vi "Init.vi"() -> (3 "Template Msg Strategy out":refnum<class "Template Msg Strategy.lvclass">)   [LabVIEW 2021, in "jettl Msg Template.lvlib" / "Template Msg Strategy.lvclass"]
uses:
  Template Msg Strategy.lvclass
  Template Msg Strategy.lvclass/Template Msg Strategy.ctl
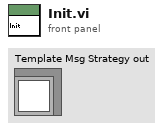
[diagram p1: front panel]
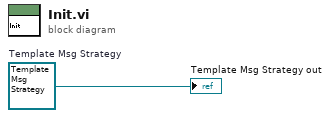
[diagram p0: block diagram]
diagram:
  w1 = refnum<class "Template Msg Strategy.lvclass"> refnum  # Template Msg Strategy
  "Template Msg Strategy out" <- w1
